vi "FreqPwrMeasureFetch.vi"(7 "Freq/Pwr":T1, 8 "error in (no error)":errorcluster) -> (0 "error out":errorcluster, 3 "FreqFetchCMD":string="FETCh:RFSA:GPRF:FCOunt:FREQuency?")   [LabVIEW 2015]
uses:
  PwrFreq.ctl
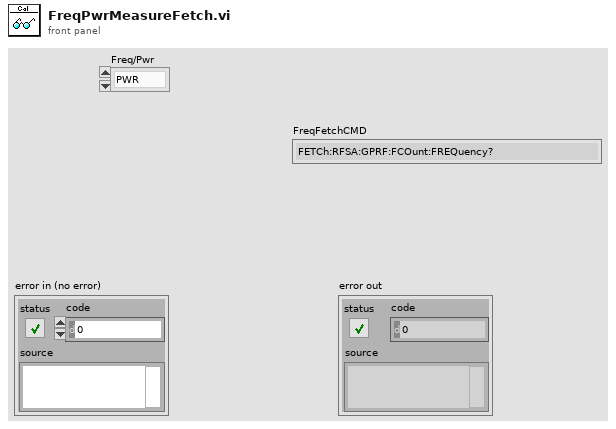
[diagram p1: front panel]
types:
  T1 = typedef "PwrFreq.ctl" = enum16{"PWR", "FREQ"}
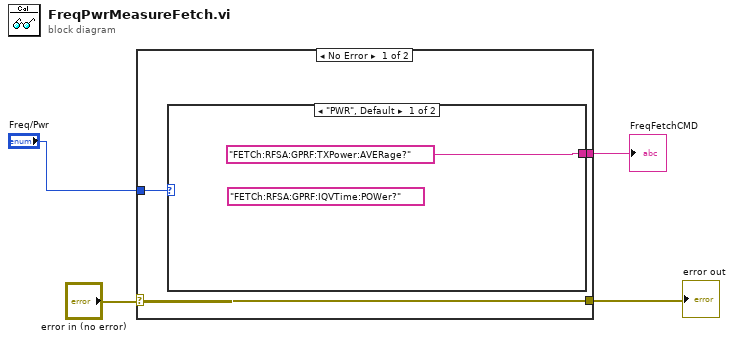
[diagram p0: block diagram]
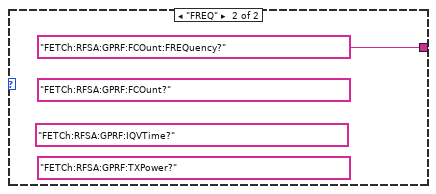
[diagram p2: hidden frame]
diagram:
  n1 = case shown="No Error" "error in (no error)" {
    selector: "error in (no error)" -> [w7 w10]
    tunnel: [w7 w10] -> w3
    tunnel: [w6 _] -> w2
    tunnel: "Freq/Pwr" -> [w5 _]
    frame No Error {
      n2 = case shown="\"PWR\", Default" w5 {
        tunnel: ["FETCh:RFSA:GPRF:TXPower:AVERage?" "FETCh:RFSA:GPRF:FCOunt:FREQuency?"] -> w6
        frame "PWR", Default {
          (unwired) "FETCh:RFSA:GPRF:IQVTime:POWer?"
        }
        frame "FREQ" {
          (unwired) "FETCh:RFSA:GPRF:TXPower?"
          (unwired) "FETCh:RFSA:GPRF:IQVTime?"
          (unwired) "FETCh:RFSA:GPRF:FCOunt?"
        }
      }
    }
    frame Error {
    }
  }
  "error out" <- w3
  "FreqFetchCMD" <- w2
